vi "Copy Array to Image (ARGB).vi"(7 "Set Alpha Values to 255 (Default: True)":bool=TRUE, 8 "error in (no error)":errorcluster, 10 "ARGB Image Destination":T1, 11 "U32 ARBG Data":u32[][](array[numeric])) -> (0 "error out":errorcluster, 3 "ARGB Image Destination (Duplicate)":T1)   [LabVIEW 2020, in "g_ar_toolkit.image.lvlib"]
uses:
  g_ar_toolkit.image.lvlib
  ARGB Image.ctl
  g_ar_toolkit.common/g_ar_toolkit.common.lvlib
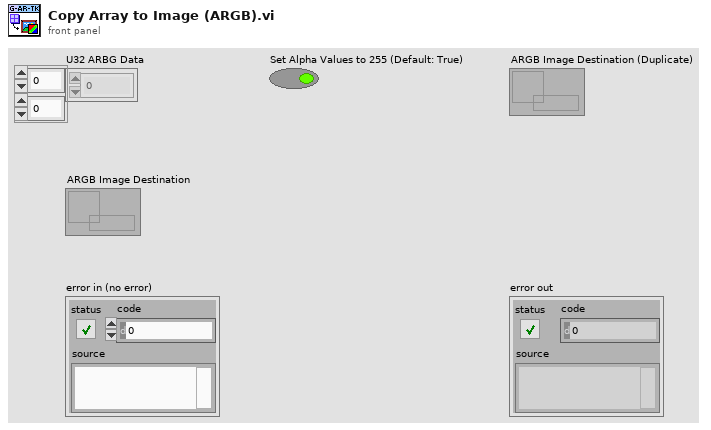
[diagram p1: front panel]
types:
  T1 = typedef "g_ar_toolkit.image.lvlib/ARGB Image.ctl" = refnum<data-value>
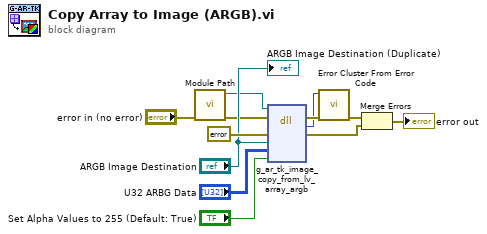
[diagram p0: block diagram]
diagram:
  n1 = call "Module Path.vi"("error in (no error)"="error in (no error)") -> ("error out"=w4:errorcluster, "Path"=w3:path)  [unwired: 9 in]
  n2 = dll-call lib="?" fn="g_ar_tk_image_copy_from_lv_array_argb" ("g_ar_toolkit.*.*:g_ar_tk_image_copy_from_raw_memory")(path in=w3, error in=w4, "error_cluster"=errorcluster {"status"=FALSE, "code"=0, "source"=""} ("error constant"), "edvr_dst"="ARGB Image Destination", "array"="U32 ARBG Data", "set_alpha_255"="Set Alpha Values to 255 (Default: True)") -> (error out=w6:errorcluster, "MgErr"=w5:i32, "error_cluster"=w11:errorcluster)  [unwired: 4 in, 1 out]
  n3 = call <vilib>:"Error Cluster From Error Code.vi"("error in (no error)"=w6, "error code (0)"=w5) -> ("error out"=w7:errorcluster)  [unwired: 7 in]
  n4 = Merge Errors(w7, w11) -> (→"error out":errorcluster)
  "ARGB Image Destination (Duplicate)" <- "ARGB Image Destination"
